vi "xy2roi.vi"(2 "ROI1":i32, 4 "xy":i32[](array[numeric]), 5 "Y Resolution":i32, 6 "X Resolution":i32) -> (0 "xy out":dbl[](array[numeric]), 1 "ROI":i32[](array[numeric]))   [LabVIEW 2011]
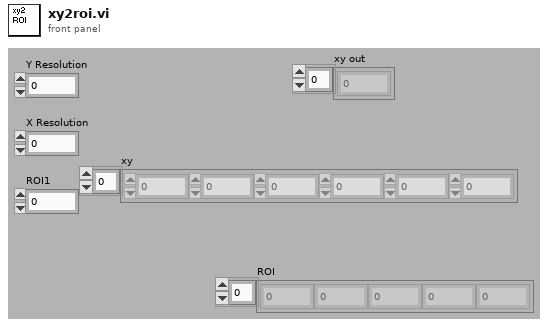
[diagram p1: front panel]
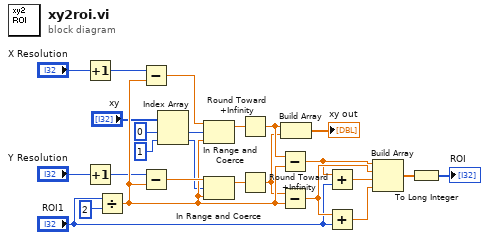
[diagram p0: block diagram]
diagram:
  n1 = Increment(x="X Resolution") -> (x+1=w19:i32)
  n2 = Increment(x="Y Resolution") -> (x+1=w10:i32)
  n3 = Divide(x="ROI1", y=2) -> (x/y=w24:dbl)
  n4 = Subtract(x=w19, y=w24) -> (x-y=w20:dbl)
  n5 = Subtract(x=w10, y=w24) -> (x-y=w25:dbl)
  n6 = Index Array(array="xy", index #1=0 ("index"), index #2=1 ("index")) -> (element #1=w5:i32, element #2=w6:i32)
  n7 = In Range and Coerce(upper limit=w20, x=w5, lower limit=w24) -> (coerced(x)=w21:dbl)  [unwired: 1 out]
  n8 = In Range and Coerce(upper limit=w25, x=w6, lower limit=w24) -> (coerced(x)=w22:dbl)  [unwired: 1 out]
  n9 = Round Toward +Infinity(x=w21) -> (ceil(x): smallest int >= x=w3:dbl)
  n10 = Round Toward +Infinity(x=w22) -> (ceil(x): smallest int >= x=w2:dbl)
  n11 = Subtract(x=w3, y=w24) -> (x-y=w12:dbl)
  n12 = Subtract(x=w2, y=w24) -> (x-y=w14:dbl)
  n13 = Build Array(w3, w2) -> (→"xy out":dbl[])
  n14 = Add(x=w12, y="ROI1") -> (x+y=w13:dbl)
  n15 = Add(x=w14, y="ROI1") -> (x+y=w15:dbl)
  n16 = Build Array(w12, w14, w13, w15) -> (w16:dbl[])
  n17 = To Long Integer(number=w16) -> (32bit integer=→"ROI":i32[])
